vi "Actor Core.vi"(8 "error in":errorcluster, 11 "ChartView In":refnum<class "ChartView.lvclass">) -> (0 "error out":errorcluster, 3 "Actor out":refnum<class "Actor.lvclass">)   [LabVIEW 2017, in "MVA Example.lvlib" / "ChartView.lvclass"]
doc: "(<B>Filename</B>: Actor Framework.lvlib:Actor.lvclass:Actor Core.vi)\n\nReceives messages to the actor, reacts to them, and initiates any error handling that may shut the actor down.\n\nDescendant classes may override this VI to append parallel tasks for the actor to complete while it handles messages. Overrides use the Call Parent Method node.\n\n<License>\nCopyright © 2017 Composed Systems, LLC | All rights reserved\nwww.composed.io\n\nAuthor: Ethan Stern <ethan.stern@composed.io>\n\nThis software is provided \"AS IS\" WITHOUT WARRANTIES, either express or implied, AND IS FOR EDUCATIONAL PURPOSES ONLY.\n</License>MVA Framework 1.6.0.31\nEthan Stern - Composed Systems\nCopyright (c) 2018, Composed Systems"
uses:
  ChartView.lvclass
  <vilib>/ActorFramework/Actor/Actor.lvclass
  <vilib>/Composed Systems/MVA Framework/Framework/IViewable/IViewable/IViewable.lvclass
panel:
  out "Waveform Chart":dbl(graph)
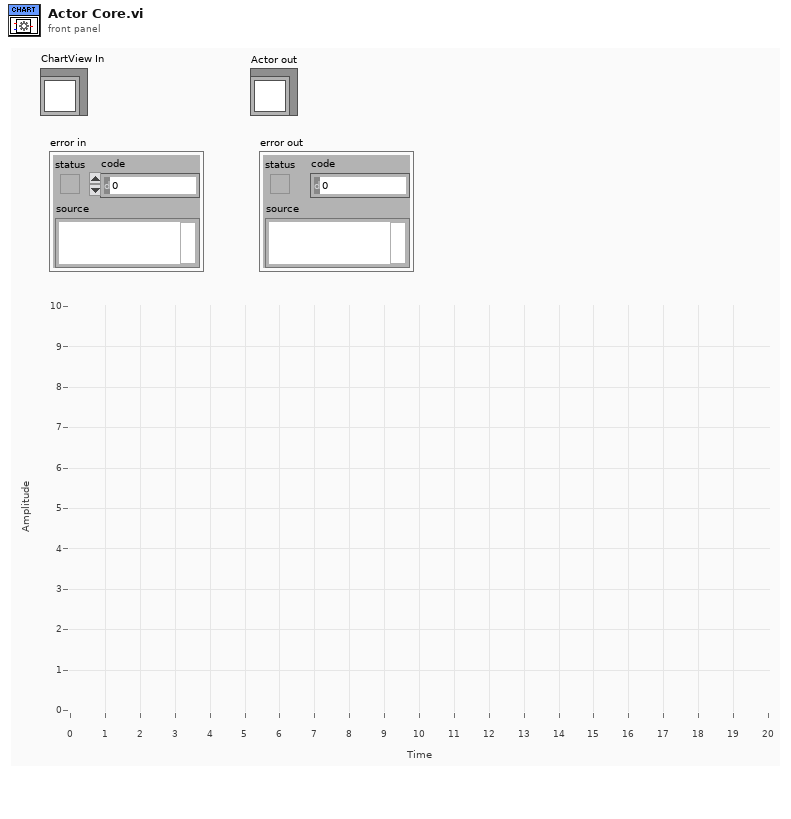
[diagram p1: front panel]
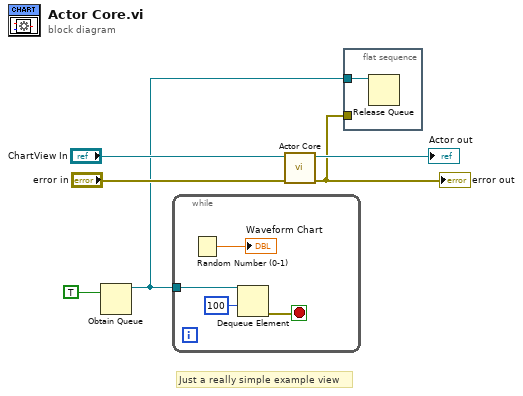
[diagram p0: block diagram]
diagram:
  # "Just a really simple example view"
  n1 = Obtain Queue(element data type=TRUE) -> (queue out=w1:refnum<queue>)  [unwired: 4 in, 2 out]
  n2 = while {
    tunnel: w1 -> [w9]
    stop <- w7 stop-if-true
    n3 = Random Number (0-1)() -> (number: 0 to 1=→"Waveform Chart":dbl)
    n4 = Dequeue Element(queue=w9, timeout in ms (-1)=100) -> (error out=w7:errorcluster)  [unwired: 1 in, 3 out]
  }
  n5 = call-parent "Actor Core.vi"("error in"="error in", "IViewable In"="ChartView In") -> ("error out"=w2:errorcluster, "Actor out"=→"Actor out":refnum<class "Actor.lvclass">)  [unwired: 8 in]
  "error out" <- w2
  n6 = flat-sequence {
    tunnel: w2 -> [_]
    tunnel: w1 -> [w11]
    frame #0 {
      n7 = Release Queue(queue=w11) -> ()  [unwired: 2 in, 3 out]
    }
  }
